vi "main_feeding.vi"(0 "Env. Ready?":refnum<vi>, 1 "Starttime":refnum<vi>, 3 "Running?":refnum<vi>, 4 "Selector":refnum<vi>, 5 "Load":refnum<vi>, 6 "Save":refnum<vi>, 7 "Valid?":refnum<vi>, 8 "New Element":refnum<vi>, 9 "Feeding":refnum<vi>, 10 "Delete":refnum<vi>, 11 "Add":refnum<vi>) -> (2 "timetable":string)   [LabVIEW 2019]
uses:
  lib/libFileFunctions/libFileFunctions.lvlib
  lib/libSimulationControl/libSimulationControl.lvlib
panel:
  out "hydro_path":path
  out "Timetable arr":string[][](array[string])
  # "*******************************************************************\nBiogas Plant Control\n\nAuthor: Paul Zügel\nGCSC-Frankfurt am Main 2020\n\n*******************************************************************"
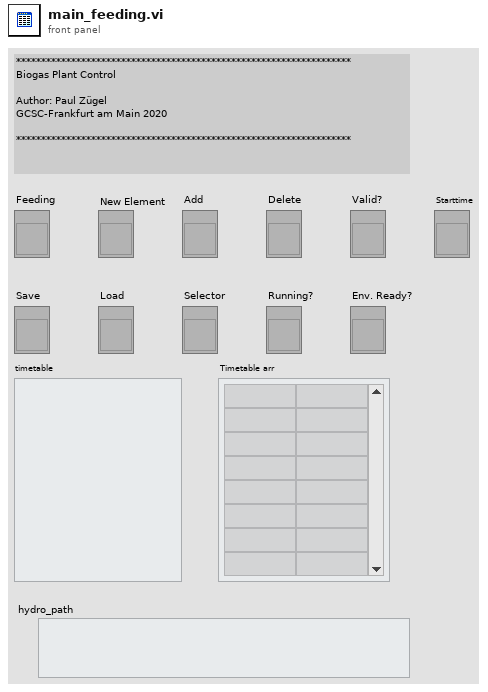
[diagram p1: front panel]
types:
  T1 = enum8{"Enabled", "Disabled", "Disabled and Grayed Out"}
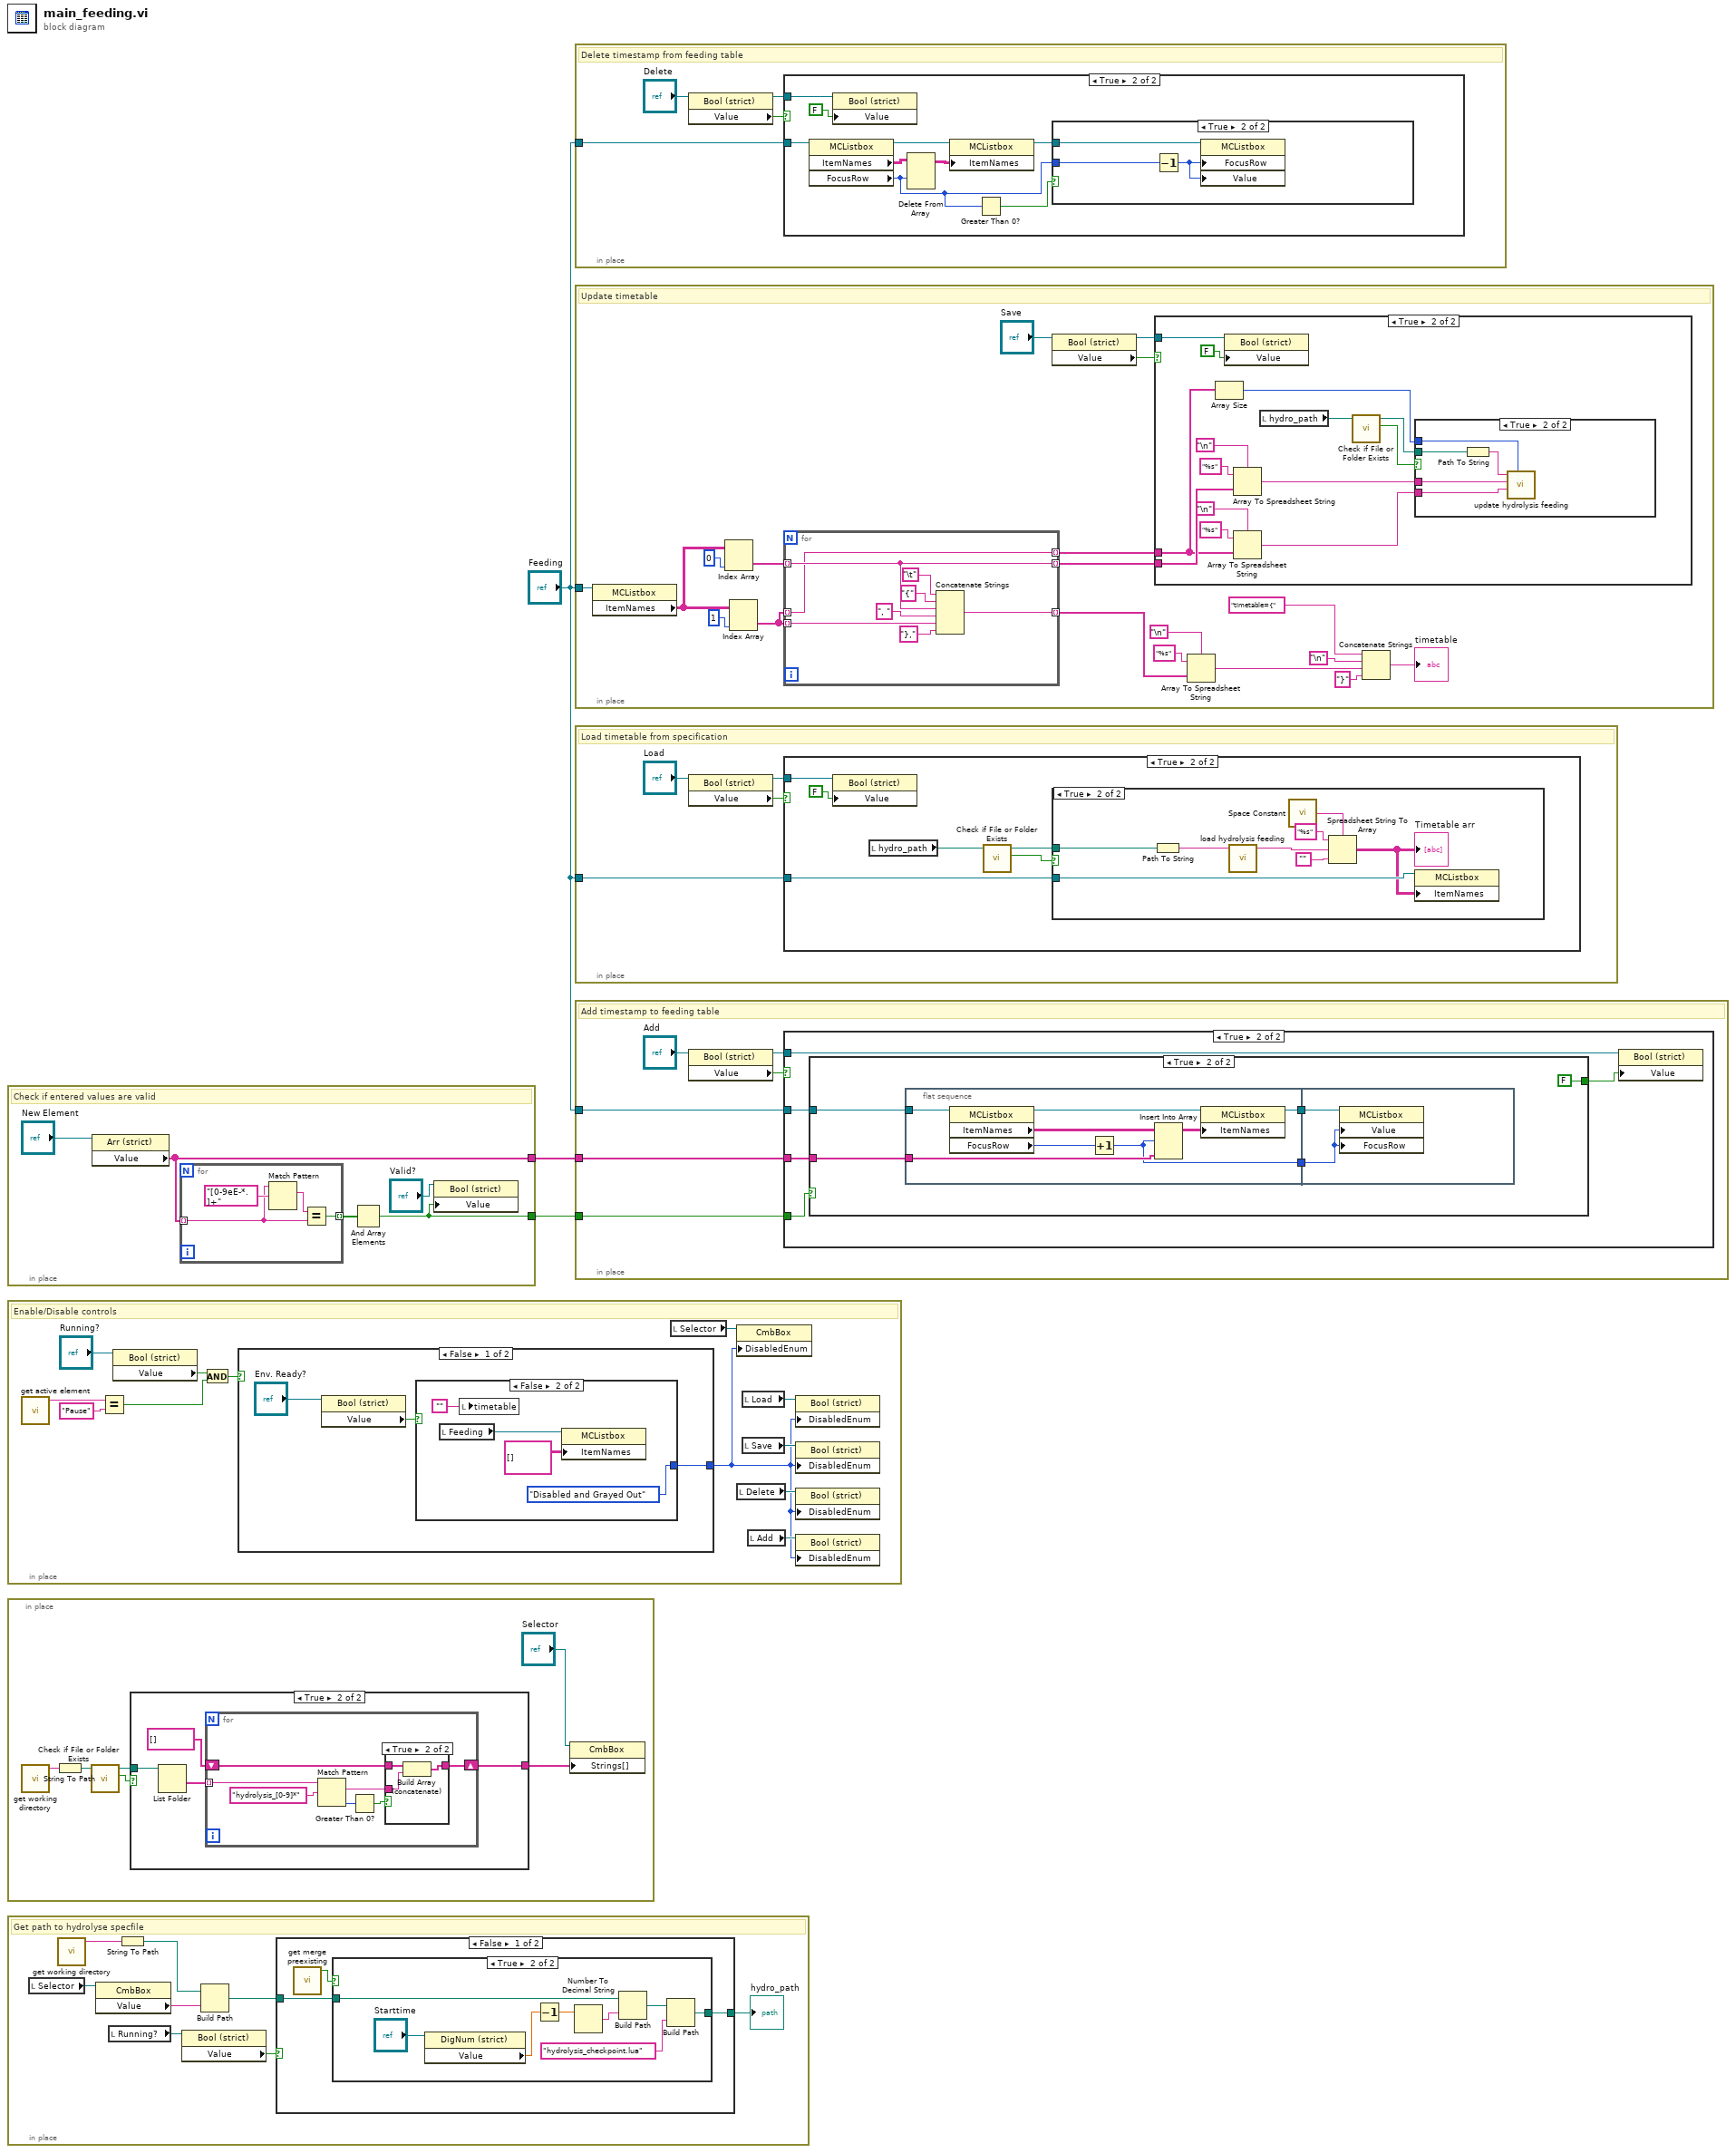
[diagram p0: block diagram]
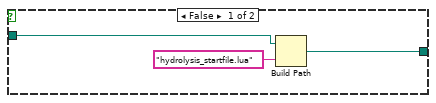
[diagram p2: hidden frame]
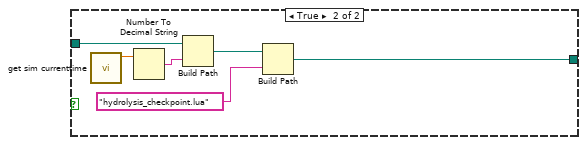
[diagram p3: hidden frame]
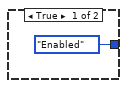
[diagram p4: hidden frame]
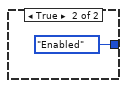
[diagram p5: hidden frame]
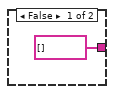
[diagram p6: hidden frame]
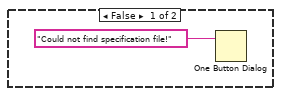
[diagram p9: hidden frame]
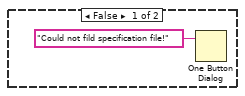
[diagram p11: hidden frame]
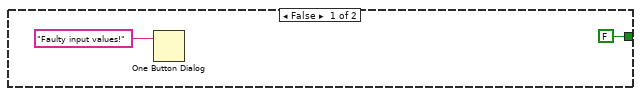
[diagram p15: hidden frame]
diagram:
  n1 = in-place {
    in-place-border: [w6] -> w3
    in-place-border: [w4] -> w2
    # "Check if entered values are valid"
    n2 = property class="Arr (strict)"(reference="New Element") -> ("Value"=w6:string[])  [unwired: 1 in, 2 out]
    n3 = for {
      tunnel: w6 -> [w10] mode=indexing
      tunnel: [w9] -> w7 mode=indexing
      n4 = Match Pattern(string=w10, regular expression="[0-9eE-*.]+") -> (match substring=w12:string)  [unwired: 1 in, 3 out]
      n5 = Equal?(x=w12, y=w10) -> (x = y?=w9:bool)
    }
    n6 = And Array Elements(Boolean array=w7) -> (logical AND=w4:bool)
    n7 = property on="Property Node" class="Bool (strict)"(reference="Valid?", "Value"=w4) -> ()  [unwired: 1 in, 2 out]
  }
  n8 = in-place {
    # "Enable/Disable controls"
    n9 = call "get active element.vi"() -> ("active_element"=w23:string)  [unwired: 10 in, 1 out]
    n10 = Equal?(x=w23, y="Pause") -> (x = y?=w20:bool)
    n11 = property class="Bool (strict)"(reference="Running?") -> ("Value"=w21:bool)  [unwired: 1 in, 2 out]
    n12 = And(x=w21, y=w20) -> (x .and. y?=w19:bool)
    n13 = case shown="False" w19 {
      tunnel: [w27 T1."Enabled" ("Disabled")] -> w13
      frame False {
        n14 = property class="Bool (strict)"(reference="Env. Ready?") -> ("Value"=w25:bool)  [unwired: 1 in, 2 out]
        n15 = case shown="False" w25 {
          tunnel: [T1."Enabled" ("Disabled") T1."Disabled and Grayed Out" ("Disabled")] -> w27
          frame True {
          }
          frame False {
            n16 = local read "Feeding"() -> (w31:refnum<vi>)
            n17 = local write "timetable"("") -> ()
            n18 = property class="MCListbox"(reference=w31, "ItemNames"=string[][] [] ("Item Names")) -> ()  [unwired: 1 in, 2 out]
          }
        }
      }
      frame True {
      }
    }
    n19 = local read "Selector"() -> (w15:refnum<vi>)
    n20 = property class="CmbBox"(reference=w15, "DisabledEnum"=w13) -> ()  [unwired: 1 in, 2 out]
    n21 = local read "Delete"() -> (w16:refnum<vi>)
    n22 = local read "Load"() -> (w17:refnum<vi>)
    n23 = local read "Save"() -> (w14:refnum<vi>)
    n24 = local read "Add"() -> (w18:refnum<vi>)
    n25 = property class="Bool (strict)"(reference=w17, "DisabledEnum"=w13) -> ()  [unwired: 1 in, 2 out]
    n26 = property class="Bool (strict)"(reference=w14, "DisabledEnum"=w13) -> ()  [unwired: 1 in, 2 out]
    n27 = property class="Bool (strict)"(reference=w16, "DisabledEnum"=w13) -> ()  [unwired: 1 in, 2 out]
    n28 = property class="Bool (strict)"(reference=w18, "DisabledEnum"=w13) -> ()  [unwired: 1 in, 2 out]
  }
  n29 = in-place {
    n30 = call "get working directory.vi"() -> ("function return"=w39:string)  [unwired: 10 in, 1 out]
    n31 = String To Path(string=w39) -> (path=w36:path)
    n32 = call <vilib>:"Check if File or Folder Exists.vi"("path"=w36) -> ("file or folder exists?"=w34:bool, "dup path"=w35:path)  [unwired: 8 in, 1 out]
    n33 = case shown="True" w34 {
      tunnel: w35 -> [_ w42]
      tunnel: [string[] [] w41] -> w37
      frame False {
      }
      frame True {
        n34 = List Folder(path=w42) -> (folder names=w44:string[])  [unwired: 3 in, 3 out]
        n35 = for {
          tunnel: w44 -> [w45] mode=indexing
          shift-right: [w46] -> w41
          shift-left: string[] [] -> [w48]
          n36 = Match Pattern(string=w45, regular expression="hydrolysis_[0-9]*") -> (match substring=w47:string, offset past match=w49:i32)  [unwired: 1 in, 2 out]
          n37 = Greater Than 0?(x=w49) -> (x > 0?=w50:bool)
          n38 = case shown="True" w50 {
            tunnel: [w52 w55] -> w46
            tunnel: w48 -> [w52 w54]
            tunnel: w47 -> [_ w53]
            frame False {
            }
            frame True {
              n39 = Build Array (concatenate)(w54, w53) -> (w55:string[])
            }
          }
        }
      }
    }
    n40 = property class="CmbBox"(reference="Selector", "Strings[]"=w37) -> ()  [unwired: 1 in, 2 out]
  }
  n41 = in-place {
    # "Get path to hydrolyse specfile"
    n42 = local read "Selector"() -> (w63:refnum<vi>)
    n43 = call "get working directory.vi"() -> ("function return"=w62:string)  [unwired: 10 in, 1 out]
    n44 = property class="CmbBox"(reference=w63) -> ("Value"=w60:string)  [unwired: 1 in, 2 out]
    n45 = local read "Running?"() -> (w57:refnum<vi>)
    n46 = String To Path(string=w62) -> (path=w61:path)
    n47 = property class="Bool (strict)"(reference=w57) -> ("Value"=w56:bool)  [unwired: 1 in, 2 out]
    n48 = Build Path(base path=w61, name or relative path=w60) -> (appended path=w59:path)
    n49 = case shown="False" w56 {
      tunnel: w59 -> [w65 w83]
      tunnel: [w64 w78] -> w58
      frame False {
        n50 = call "get merge preexisting.vi"() -> ("function return"=w66:bool)  [unwired: 10 in, 1 out]
        n51 = case shown="True" w66 {
          tunnel: w65 -> [w68 w75]
          tunnel: [w67 w74] -> w64
          frame False {
            n52 = Build Path(base path=w68, name or relative path="hydrolysis_startfile.lua") -> (appended path=w67:path)
          }
          frame True {
            n53 = property on="Property Node" class="DigNum (strict)"(reference="Starttime") -> ("Value"=w72:dbl)  [unwired: 1 in, 2 out]
            n54 = Decrement(x=w72) -> (x-1=w70:dbl)
            n55 = Number To Decimal String(number=w70) -> (decimal integer string=w71:string)  [unwired: 1 in]
            n56 = Build Path(base path=w75, name or relative path=w71) -> (appended path=w77:path)
            n57 = Build Path(base path=w77, name or relative path="hydrolysis_checkpoint.lua") -> (appended path=w74:path)
          }
        }
      }
      frame True {
        n58 = call "get sim currenttime.vi"() -> ("current_time"=w82:dbl)  [unwired: 10 in, 1 out]
        n59 = Number To Decimal String(number=w82) -> (decimal integer string=w81:string)  [unwired: 1 in]
        n60 = Build Path(base path=w83, name or relative path=w81) -> (appended path=w80:path)
        n61 = Build Path(base path=w80, name or relative path="hydrolysis_checkpoint.lua") -> (appended path=w78:path)
      }
    }
    "hydro_path" <- w58
  }
  n62 = in-place {
    in-place-border: "Feeding" -> [w87]
    # "Delete timestamp from feeding table"
    n63 = property on="Property Node" class="Bool (strict)"(reference="Delete") -> (reference out=w86:refnum<vi>, "Value"=w85:bool)  [unwired: 1 in, 1 out]
    n64 = case shown="True" w85 {
      tunnel: w87 -> [_ w96]
      tunnel: w86 -> [_ w94]
      frame False {
      }
      frame True {
        n65 = property on="Property Node" class="MCListbox"(reference=w96) -> (reference out=w91:refnum<vi>, "ItemNames"=w93:string[][], "FocusRow"=w89:i32)  [unwired: 1 in, 1 out]
        n66 = property on="Property Node" class="Bool (strict)"(reference=w94, "Value"=FALSE) -> ()  [unwired: 1 in, 2 out]
        n67 = Delete From Array(array=w93, index (row)=w89) -> (array with subset deleted=w92:string[][])  [unwired: 2 in, 1 out]
        n68 = property on="Property Node" class="MCListbox"(reference=w91, "ItemNames"=w92) -> (reference out=w95:refnum<vi>)  [unwired: 1 in, 1 out]
        n69 = Greater Than 0?(x=w89) -> (x > 0?=w88:bool)
        n70 = case shown="True" w88 {
          tunnel: w89 -> [_ w99]
          tunnel: w95 -> [_ w98]
          frame False {
          }
          frame True {
            n71 = Decrement(x=w99) -> (x-1=w97:i32)
            n72 = property on="Property Node" class="MCListbox"(reference=w98, "FocusRow"=w97, "Value"=w97) -> ()  [unwired: 1 in, 2 out]
          }
        }
      }
    }
  }
  n73 = in-place {
    in-place-border: "Feeding" -> [w111]
    # "Update timetable"
    n74 = property on="Property Node" class="MCListbox"(reference=w111) -> ("ItemNames"=w112:string[][])  [unwired: 1 in, 2 out]
    n75 = Index Array(array=w112, index (col)=0 ("disabled index (col)")) -> (element=w114:string[])  [unwired: 1 in]
    n76 = Index Array(array=w112, index (col)=1 ("disabled index (col)")) -> (element=w102:string[])  [unwired: 1 in]
    n77 = for {
      tunnel: w114 -> [w140] mode=indexing
      tunnel: w102 -> [w141] mode=indexing
      tunnel: [w146] -> w113 mode=indexing
      tunnel: [w139] -> w103 mode=indexing
      tunnel: [w140] -> w101 mode=indexing
      tunnel: w102 -> [w139] mode=indexing
      n78 = Concatenate Strings("\t", "{" ("string"), w140, ", " ("string"), w141, "}," ("string")) -> (w146:string)
    }
    n79 = property class="Bool (strict)"(reference="Save") -> (reference out=w100:refnum<vi>, "Value"=w105:bool)  [unwired: 1 in, 1 out]
    n80 = case shown="True" w105 {
      tunnel: w103 -> [_ w125]
      tunnel: w101 -> [_ w131]
      tunnel: w100 -> [_ w123]
      frame False {
      }
      frame True {
        n81 = Array Size(array=w125) -> (size(s)=w132:i32)
        n82 = property class="Bool (strict)"(reference=w123, "Value"=FALSE) -> ()  [unwired: 1 in, 2 out]
        n83 = Array To Spreadsheet String(delimiter (Tab)="\n", array=w131, 3:"%s" ("format string")) -> (spreadsheet string=w128:string)
        n84 = Array To Spreadsheet String(delimiter (Tab)="\n", array=w125, 3:"%s" ("format string")) -> (spreadsheet string=w124:string)
        n85 = local read "hydro_path"() -> (w121:path)
        n86 = call <vilib>:"Check if File or Folder Exists.vi"("path"=w121) -> ("file or folder exists?"=w120:bool, "dup path"=w119:path)  [unwired: 8 in, 1 out]
        n87 = case shown="True" w120 {
          tunnel: w132 -> [_ w138]
          tunnel: w128 -> [_ w137]
          tunnel: w124 -> [_ w136]
          tunnel: w119 -> [_ w135]
          frame False {
            n88 = One Button Dialog(message="Could not fild specification file!") -> ()  [unwired: 1 in, 1 out]
          }
          frame True {
            n89 = Path To String(path=w135) -> (string=w134:string)
            n90 = call "update hydrolysis feeding.vi"("number_timestamps"=w138, "amount"=w136, "time"=w137, "hydrolysis_specfile"=w134) -> ()  [unwired: 7 in, 1 out]
          }
        }
      }
    }
    n91 = Array To Spreadsheet String(delimiter (Tab)="\n", array=w113, 3:"%s" ("format string")) -> (spreadsheet string=w108:string)
    n92 = Concatenate Strings("timetable={" ("string"), "\n", w108, "}" ("string")) -> (→"timetable":string)
  }
  n93 = in-place {
    in-place-border: "Feeding" -> [w150]
    # "Load timetable from specification"
    n94 = property on="Property Node" class="Bool (strict)"(reference="Load") -> (reference out=w147:refnum<vi>, "Value"=w148:bool)  [unwired: 1 in, 1 out]
    n95 = case shown="True" w148 {
      tunnel: w150 -> [_ w156]
      tunnel: w147 -> [_ w155]
      frame False {
      }
      frame True {
        n96 = property on="Property Node" class="Bool (strict)"(reference=w155, "Value"=FALSE) -> ()  [unwired: 1 in, 2 out]
        n97 = local read "hydro_path"() -> (w153:path)
        n98 = call <vilib>:"Check if File or Folder Exists.vi"("path"=w153) -> ("file or folder exists?"=w152:bool, "dup path"=w151:path)  [unwired: 8 in, 1 out]
        n99 = case shown="True" w152 {
          tunnel: w156 -> [_ w165]
          tunnel: w151 -> [_ w159]
          frame False {
            n100 = One Button Dialog(message="Could not find specification file!") -> ()  [unwired: 1 in, 1 out]
          }
          frame True {
            n101 = Path To String(path=w159) -> (string=w158:string)
            n102 = call "load hydrolysis feeding.vi"("hydrolysis_specfile"=w158) -> ("function return"=w164:string)  [unwired: 9 in, 1 out]
            n103 = call <vilib>:"Space Constant.vi"() -> ("String"=w160:string)
            n104 = Spreadsheet String To Array(delimiter (Tab)=w160, format string="%s", spreadsheet string=w164, array type (2D Dbl)="") -> (array=w161:string[][])
            "Timetable arr" <- w161
            n105 = property class="MCListbox"(reference=w165, "ItemNames"=w161) -> ()  [unwired: 1 in, 2 out]
          }
        }
      }
    }
  }
  n106 = in-place {
    in-place-border: "Feeding" -> [w171]
    in-place-border: w3 -> [w168]
    in-place-border: w2 -> [w167]
    # "Add timestamp to feeding table"
    n107 = property class="Bool (strict)"(reference="Add") -> (reference out=w169:refnum<vi>, "Value"=w170:bool)  [unwired: 1 in, 1 out]
    n108 = case shown="True" w170 {
      tunnel: w171 -> [_ w176]
      tunnel: w169 -> [_ w174]
      tunnel: w168 -> [_ w173]
      tunnel: w167 -> [_ w172]
      frame False {
      }
      frame True {
        n109 = case shown="True" w172 {
          tunnel: w173 -> [_ w183]
          tunnel: w176 -> [_ w181]
          tunnel: [FALSE ("Value") FALSE ("Value")] -> w175
          frame False {
            n110 = One Button Dialog(message="Faulty input values!") -> ()  [unwired: 1 in, 1 out]
          }
          frame True {
            n111 = flat-sequence {
              tunnel: w183 -> [w191]
              tunnel: [w188] -> w182
              tunnel: w181 -> [w186]
              tunnel: [w184] -> w180
              tunnel: w182 -> [w193]
              tunnel: w180 -> [w192]
              frame #0 {
                n112 = property on="Property Node" class="MCListbox"(reference=w186) -> (reference out=w185:refnum<vi>, "ItemNames"=w190:string[][], "FocusRow"=w187:i32)  [unwired: 1 in, 1 out]
                n113 = Increment(x=w187) -> (x+1=w188:i32)
                n114 = Insert Into Array(array=w190, index (row)=w188, new element=w191) -> (w189:string[][])  [unwired: 1 in]
                n115 = property on="Property Node" class="MCListbox"(reference=w185, "ItemNames"=w189) -> (reference out=w184:refnum<vi>)  [unwired: 1 in, 1 out]
              }
              frame #1 {
                n116 = property on="Property Node" class="MCListbox"(reference=w192, "Value"=w193, "FocusRow"=w193) -> ()  [unwired: 1 in, 2 out]
              }
            }
          }
        }
        n117 = property class="Bool (strict)"(reference=w174, "Value"=w175) -> ()  [unwired: 1 in, 2 out]
      }
    }
  }
